vi "hemholtz_analyzer.vi"() -> ()   [LabVIEW 2023]
uses:
  <vilib>/express/express analysis/Spectral/Block/exnSpectralBlock spectral measurements RMS poly.vi
  <vilib>/express/express analysis/Spectral/Block/exnSpectralBlock spectral measurements RMS DDT.vi
  <vilib>/measure/matone.llb/Extract Single Tone Information N Chan.vi
  <vilib>/express/express analysis/Spectral/XNode/ExpressSpectralMeasurementsBlockNode.xnode
  <vilib>/measure/NI_MAPro.lvlib
panel:
  in  "Duration (s)":dbl=1.0
  out "Detected Frequency":dbl[](array[numeric]) format="%.2p"
  out "Expected Frequency":dbl
  in  "h":dbl
  in  "h_j":dbl
  in  "h_t":dbl
  in  "d_j":dbl
  in  "d_t":dbl
  out "Waveform Graph":dynamicdata(graph)
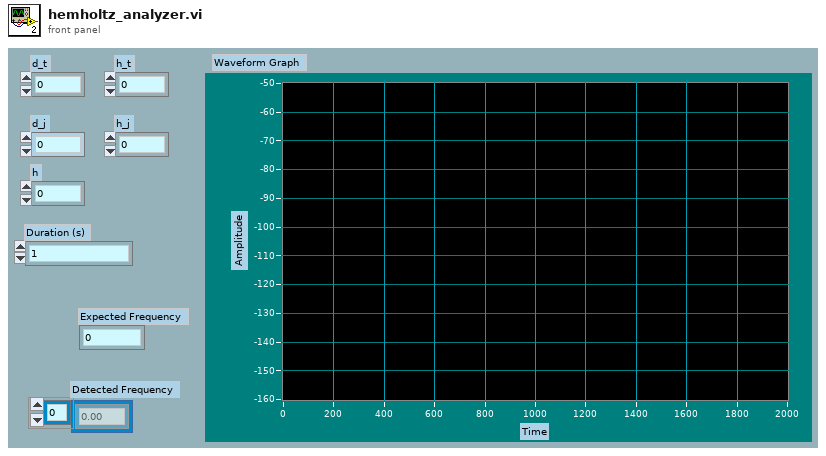
[diagram p1: front panel]
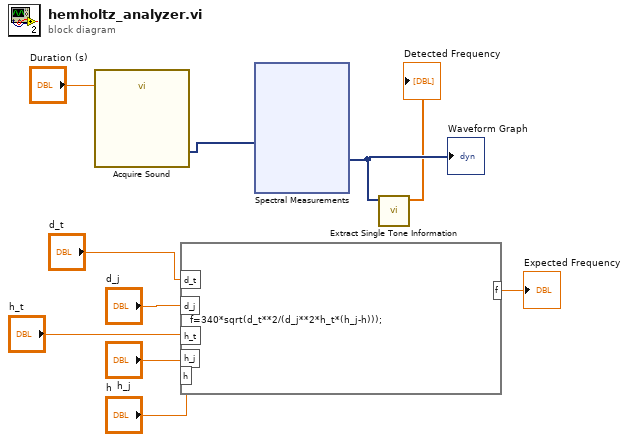
[diagram p0: block diagram]
diagram:
  n1 = call "Acquire Sound"("Duration (s)"="Duration (s)") -> ("Data"=w10:dynamicdata)  [unwired: 17 in, 1 out]
  n2 = formula code="f=340*sqrt(d_t**2/(d_j**2*h_t*(h_j-h)));"("d_t"="d_t", "d_j"="d_j", "h_t"="h_t", "h_j"="h_j", "h"="h") -> ("f"=→"Expected Frequency":dbl)
  n3 = xnode "Spectral Measurements"("Signals"=w10) -> ("FFT - (RMS)"=w3:dynamicdata)  [unwired: 1 in, 2 out]
  "Waveform Graph" <- w3
  n4 = call-poly <vilib>:"Extract Single Tone Information.vi"("time signals in"=w3) -> ("detected frequencies"=→"Detected Frequency":dbl[])  [unwired: 5 in, 5 out]
